vi "Configure Bandwidth Part.vi"(0 "VISA resource name":refnum<visa-resource-name>, 1 "Subcarrier Spacing (15 kHz)":i32(ring) items=["15 kHz", "30 kHz", "60 kHz"], 2 "No Of RBs (50)":i32=50, 5 "Instance (1)":T2=1, 7 "CC (1)":T1=1, 9 "BWP (BWP0)":i32(ring) items=["BWP0"], 11 "error in (no error)":errorcluster, 12 "Cyclic Prefix (Normal)":i32(ring) items=["Normal", "Extended"], 13 "Start RB (0)":i32) -> (4 "VISA resource name out":refnum<visa-resource-name>, 15 "error out":errorcluster)   [LabVIEW 2020, in "Rohde&Schwarz CMWXP NR FR1 Measurement.lvlib"]
doc: "Configures basic properties of the <BWP> on carrier <CC>.\n\nAttribute:\nRSCMWXPNRFR1M_ATTR_BANDWIDTH_PART\n\nRemote-control command:\nCONFigure:NRSub:MEAS<i>[:CC<no>]:BWPart"
uses:
  <instrlib>/Rohde&Schwarz CMWXP NR FR1 Measurement/Rohde&Schwarz CMWXP NR FR1 Measurement.lvlib
  <instrlib>/Rohde&Schwarz CMWXP NR FR1 Measurement/Private/_Instance.ctl
  <instrlib>/Rohde&Schwarz CMWXP NR FR1 Measurement/Private/_Carrier Component.ctl
  <instrlib>/Rohde&Schwarz CMWXP NR FR1 Measurement/Private/rsidr_core.llb/rsidr_core.lvlib
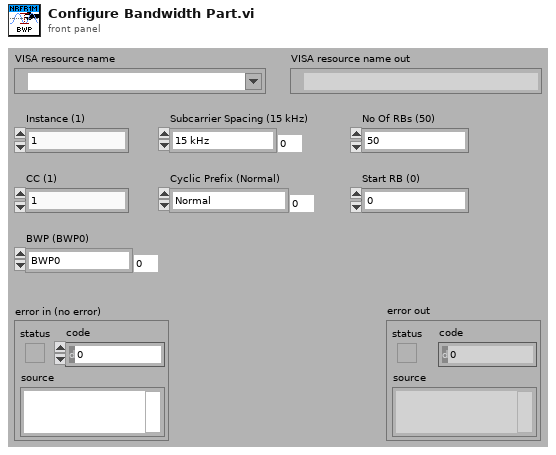
[diagram p1: front panel]
types:
  T1 = typedef "Rohde&Schwarz CMWXP NR FR1 Measurement.lvlib/_Carrier Component.ctl" = i32
  T2 = typedef "Rohde&Schwarz CMWXP NR FR1 Measurement.lvlib/_Instance.ctl" = i32
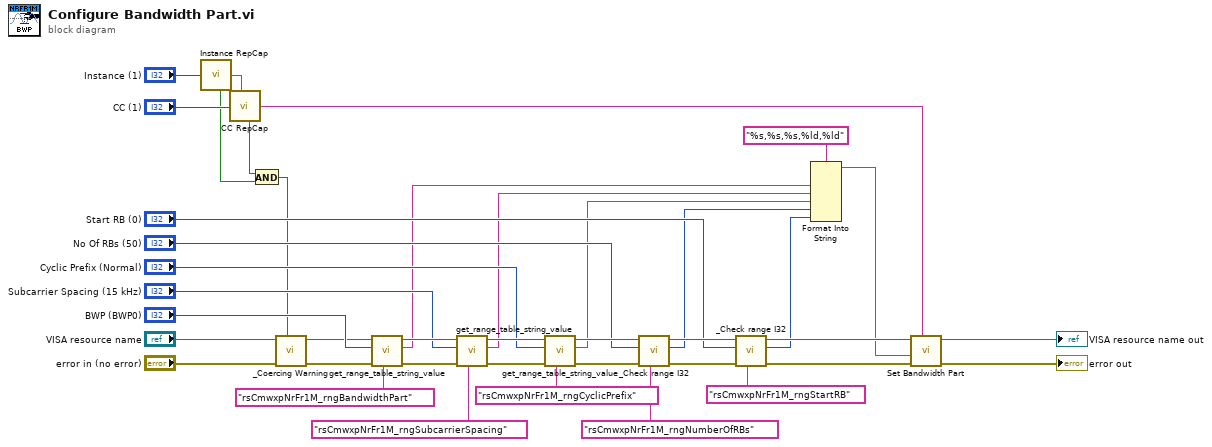
[diagram p0: block diagram]
diagram:
  n1 = call <instrlib>:"Instance RepCap.vi"("Instance In"="Instance (1)") -> ("In Range?"=w1:bool, "RepCap Identifier Out"=w38:string)  [unwired: 1 in]
  n2 = call <instrlib>:"CC RepCap.vi"("CC In"="CC (1)", "RepCap String In (\"\")"=w38) -> ("In Range?"=w2:bool, "RepCap Identifier Out"=w15:string)
  n3 = And(x=w2, y=w1) -> (x .and. y?=w3:bool)
  n4 = call <instrlib>:"_Coercing Warning.vi"("In Range?"=w3, "error in (no error)"="error in (no error)", "VISA resource name"="VISA resource name") -> ("error out"=w5:errorcluster, "VISA resource name out"=w4:refnum<visa-resource-name>)  [unwired: 7 in]
  n5 = call <instrlib>:"get_range_table_string_value.vi"("Range Table ID in"="rsCmwxpNrFr1M_rngBandwidthPart", "error in"=w5, "I32 input"="BWP (BWP0)", "VISA resource name"=w4) -> ("error out"=w37:errorcluster, "String Value out"=w13:string, "VISA resource name out"=w36:refnum<visa-resource-name>)  [unwired: 5 in]
  n6 = call <instrlib>:"get_range_table_string_value.vi"("Range Table ID in"="rsCmwxpNrFr1M_rngSubcarrierSpacing", "error in"=w37, "I32 input"="Subcarrier Spacing (15 kHz)", "VISA resource name"=w36) -> ("error out"=w35:errorcluster, "String Value out"=w12:string, "VISA resource name out"=w34:refnum<visa-resource-name>)  [unwired: 5 in]
  n7 = call <instrlib>:"get_range_table_string_value.vi"("Range Table ID in"="rsCmwxpNrFr1M_rngCyclicPrefix", "error in"=w35, "I32 input"="Cyclic Prefix (Normal)", "VISA resource name"=w34) -> ("error out"=w33:errorcluster, "String Value out"=w11:string, "VISA resource name out"=w32:refnum<visa-resource-name>)  [unwired: 5 in]
  n8 = call <instrlib>:"_Check range I32.vi"("Range Table Identifier"="rsCmwxpNrFr1M_rngNumberOfRBs", "error in (no error)"=w33, "I32 Value In"="No Of RBs (50)", "VISA resource name"=w32) -> ("error out"=w31:errorcluster, "I32 Value Out"=w10:i32, "VISA resource name out"=w30:refnum<visa-resource-name>)  [unwired: 5 in]
  n9 = call <instrlib>:"_Check range I32.vi"("Range Table Identifier"="rsCmwxpNrFr1M_rngStartRB", "error in (no error)"=w31, "I32 Value In"="Start RB (0)", "VISA resource name"=w30) -> ("error out"=w29:errorcluster, "I32 Value Out"=w9:i32, "VISA resource name out"=w26:refnum<visa-resource-name>)  [unwired: 5 in]
  n10 = Format Into String(format string="%s,%s,%s,%ld,%ld", w13, w12, w11, w10, w9) -> (resulting string=w8:string)  [unwired: 2 in, 1 out]
  n11 = call "Set Bandwidth Part"("Repeated Capabilities"=w15, "error in (no error)"=w29, "Bandwidth Part ()"=w8, "instrument handle"=w26) -> ("error out"=→"error out":errorcluster, "instrument handle out"=→"VISA resource name out":refnum<visa-resource-name>)  [unwired: 6 in]
